vi "ZoomImage.vi"(11 "XY Shifts":dbl[](array[numeric])) -> (3 "Inner Crop Rect":dbl[](array[numeric]))   [LabVIEW 2020]
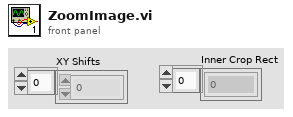
[diagram p1: front panel]
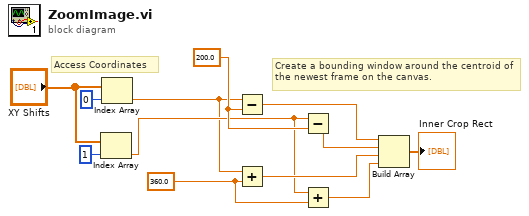
[diagram p0: block diagram]
diagram:
  w7 = 200.0 ("y")
  w10 = 360.0 ("y")
  # "Create a bounding window around the centroid of the newest frame on the canvas."
  # "Access Coordinates"
  n1 = Index Array(array="XY Shifts", index=1) -> (element=w5:dbl)
  n2 = Index Array(array="XY Shifts", index=0) -> (element=w2:dbl)
  n3 = Subtract(x=w2, y=w7) -> (x-y=w6:dbl)
  n4 = Add(x=w2, y=w10) -> (x+y=w9:dbl)
  n5 = Subtract(x=w5, y=w7) -> (x-y=w4:dbl)
  n6 = Add(x=w5, y=w10) -> (x+y=w8:dbl)
  n7 = Build Array(w6, w4, w9, w8) -> (→"Inner Crop Rect":dbl[])
